vi "Example_OE1311&1351 Ethernet_Query Setting.vi"() -> ()   [LabVIEW 2011]
panel:
  in  "Ethernet":T1={"Port"=10001, "Timeout"=1000, "IP Address"=""}
  out "System":T2
  out "Sensitivity and Filter":T3={"Input Range"=2, "Time Constant(s) "=[], "Low Pass Filter Slope "=1, "Enable Sync Filter "=0} {"Enable Sync Filter" items=["OFF", "ON"]; "Low Pass Filter Slope" items=["6 dB/oct", "12 dB/oct", "18 db/oct", "24 dB/oct", "30 dB/oct", "36 dB/oct", "42 dB/oct", "48 dB/oct"]; "Input Range" items=["5 V/uA", "2 V/uA", "1 V/uA", "500 mV/nA", "200 mV/nA", "100 mV/nA", "50 mV/nA", "20 mV/nA", "10 mV/nA", "5 mV/nA", "2 mV/nA", "1 mV/nA", "500 uV/pA", "200 uV/pA", "100 uV/pA", "50 uV/pA", "20 uV/pA", "10 uV/pA", "5 uV/pA", "2 uV/pA", "1 uV/pA", "500 nV/fA", "200 nV/fA", "100 nV/fA", "50 nV/fA", "20 nV/fA", "10 nV/fA", "5 nV/fA", "2 nV/fA", "1 nV/fA"]}
  out "Sine Out":T4 {"SineOut Mode" items=["OFF", "Fixed"]}
  out "Channel Out":T5={"Ch_source_1"=3, "Ch_source_2"=3, "AUX OUT1"=[], "AUX OUT2"=[], "CH1 Offset(%)"=[], "CH2 Offset(%)"=[], "CH1 Expand"=[], "CH2 Expand"=[]} {"Ch_source_2" items=["Fixed", "X", "Y", "R", "Theta", "Xh1", "Yh1", "Rh1", "Theta h1", "Xh2", "Yh2", "Rh2", "Theta h2", "Xh3", "Yh3", "Rh3", "Theta h3", "Rh4", "Xh4", "Yh4", "Theta h4", "Rh5", "Xh5", "Yh5", "Theta h5", "Rh6", "Xh6", "Yh6", "Theta h6", "Rh7", "Xh6", "Yh6", "Theta h7", "X_Noise", "Y_Noise", "Freq", "AuxIn1", "AuxIn2"]; "Ch_source_1" items=["Fixed", "X", "Y", "R", "Theta", "Xh1", "Yh1", "Rh1", "Theta h1", "Xh2", "Yh2", "Rh2", "Theta h2", "Xh3", "Yh3", "Rh3", "Theta h3", "Rh4", "Xh4", "Yh4", "Theta h4", "Rh5", "Xh5", "Yh5", "Theta h5", "Rh6", "Xh6", "Yh6", "Theta h6", "Rh7", "Xh6", "Yh6", "Theta h7", "X_Noise", "Y_Noise", "Freq", "AuxIn1", "AuxIn2"]}
  out "Reference Phase":T6 {"External Ref Trigger" items=["TTL Rising Edge", "TTL Fallling Edge", "Sine Zero Crossing"]; "Reference Source" items=["External", "Internal", "Self"]}
  out "Demodulator":T7 {"Demodulator type_7" items=["Harm", "Arb_Freq"]; "Demodulator type_6" items=["Harm", "Arb_Freq"]; "Demodulator type_5" items=["Harm", "Arb_Freq"]; "Demodulator type_4" items=["Harm", "Arb_Freq"]; "Demodulator type_3" items=["Harm", "Arb_Freq"]; "Demodulator type_2" items=["Harm", "Arb_Freq"]; "Demodulator type_1" items=["Harm", "Arb_Freq"]}
  out "Input Filter":cluster{"InputCoupling":u8, "InputSource":u8} {"InputSource" items=["A", "B", "Current"]; "InputCoupling" items=["AC", "DC"]}
  in  "error in (no error)":errorcluster
  out "Error out":errorcluster caption="error out"
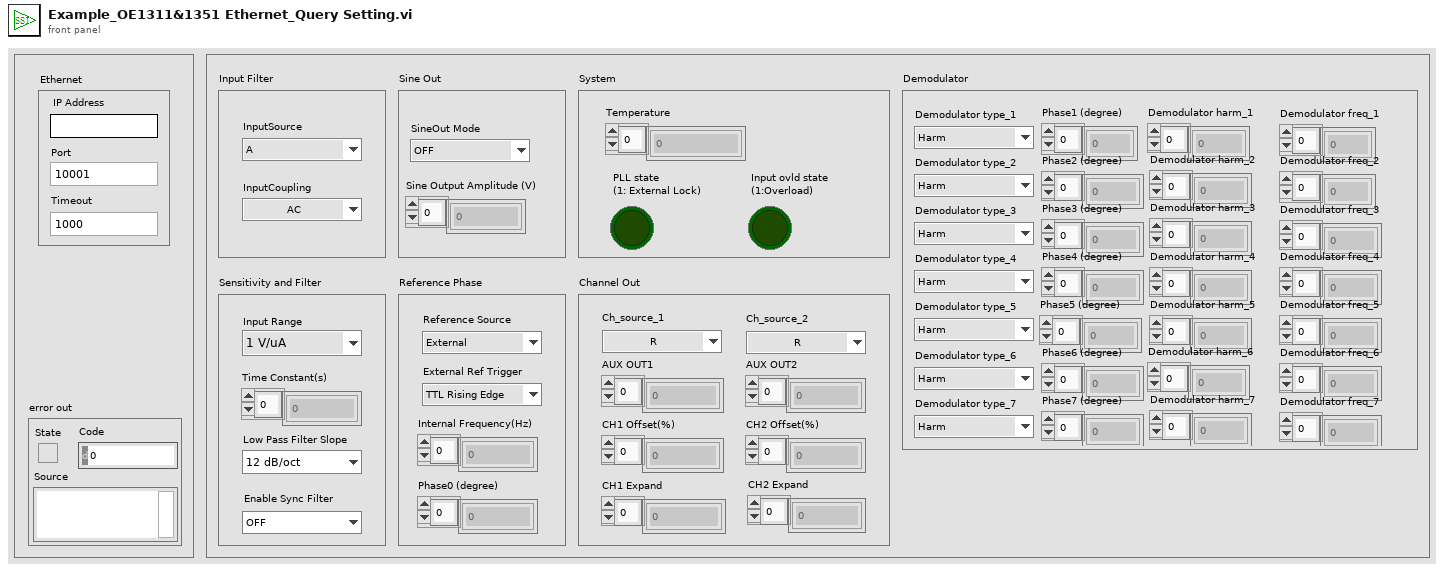
[diagram p1: front panel]
types:
  T1 = cluster{"Port":u32, "Timeout":u32, "IP Address":string}
  T2 = cluster{"Temperature":dbl[], "PLL state\n(1: External Lock)":bool, "Input ovld state\n(1:Overload)":bool}
  T3 = cluster{"Input Range":u8, "Time Constant(s) ":dbl[], "Low Pass Filter Slope ":u8, "Enable Sync Filter ":u8}
  T4 = cluster{"SineOut Mode":u8, "Sine Output Amplitude (V)":dbl[]}
  T5 = cluster{"Ch_source_1":u8, "Ch_source_2":u8, "AUX OUT1":dbl[], "AUX OUT2":dbl[], "CH1 Offset(%)":dbl[], "CH2 Offset(%)":dbl[], "CH1 Expand":dbl[], "CH2 Expand":dbl[]}
  T6 = cluster{"Phase0 (degree)":dbl[], "Internal Frequency(Hz)":dbl[], "Reference Source":u8, "External Ref Trigger":u8}
  T7 = cluster{"Demodulator type_1":u8, "Demodulator type_2":u8, "Demodulator type_3":u8, "Demodulator type_4":u8, "Demodulator type_5":u8, "Demodulator type_6":u8, "Demodulator type_7":u8, "Phase1 (degree)":dbl[], "Phase2 (degree)":dbl[], "Phase3 (degree)":dbl[], "Phase4 (degree)":sgl[], "Phase5 (degree)":dbl[], "Phase6 (degree)":dbl[], "Phase7 (degree)":dbl[], "Demodulator harm_1":u8[], "Demodulator harm_2":u8[], "Demodulator harm_3":u8[], "Demodulator harm_4":u8[], "Demodulator harm_5":u8[], "Demodulator harm_6":u8[], "Demodulator harm_7":u8[], "Demodulator freq_1":dbl[], "Demodulator freq_2":dbl[], "Demodulator freq_3":dbl[], "Demodulator freq_4":dbl[], "Demodulator freq_5":dbl[], "Demodulator freq_6":dbl[], "Demodulator freq_7":dbl[]}
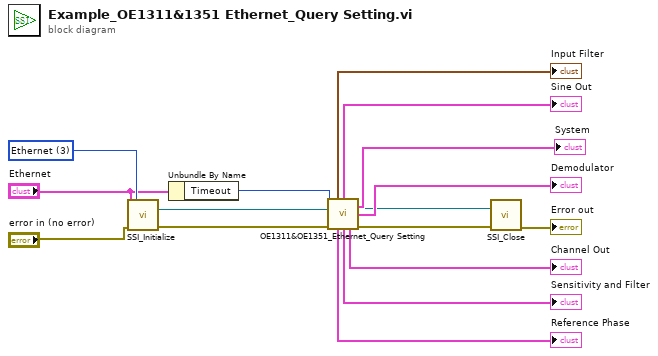
[diagram p0: block diagram]
diagram:
  w8 = u16 3 items=["USB", "RS232", "GPIB", "Ethernet"] ("Remote Mode")
  n1 = call "SSI_Initialize.vi"("Remote Mode"=w8, "Ethernet"="Ethernet", "error in (no error)"="error in (no error)") -> ("connection ID(Ethernet)"=w4:refnum<k5>, "error out"=w3:errorcluster)  [unwired: 10 in, 1 out]
  n2 = Unbundle By Name("Ethernet") -> ("Timeout"=w5:u32)
  n3 = call "OE1311&OE1351_Ethernet_Query Setting.vi"("Connection ID in"=w4, "Timeout"=w5, "Error in (no error)"=w3) -> ("Input Filter"=→"Input Filter":cluster{"InputCoupling":u8, "InputSource":u8}, "Sine Out"=→"Sine Out":T4, "System"=→"System":T2, "Connection ID out"=w1:refnum<k5>, "Demodulator"=→"Demodulator":T7, "Reference Phase"=→"Reference Phase":T6, "Sensitivity and Filter"=→"Sensitivity and Filter":T3, "Channel Out"=→"Channel Out":T5, "Error out"=w2:errorcluster)  [unwired: 3 in, 1 out]
  n4 = call "SSI_Close.vi"("Error in (no error)"=w2, "Connection ID in"=w1) -> ("Error out"=→"Error out":errorcluster)  [unwired: 5 in]
